vi "Test IODIR Configured as Output on Create.vi"(11 "Test Case In":refnum<class "MCP23017 Test.lvclass">) -> (0 "error out":errorcluster, 3 "Test Case Out":refnum<class "MCP23017 Test.lvclass">)   [LabVIEW 2020, in "MCP23017 Test.lvclass"]
uses:
  MCP23017 Test.lvclass
  C:/Program Files (x86)/National Instruments/LabVIEW 2020/vi.lib/Astemes/LUnit/Test Case.lvclass
  Mock I2C Bus/Mock I2C Bus.lvclass
  C:/Program Files (x86)/National Instruments/LabVIEW 2020/vi.lib/Astemes/LMock/Mock.lvclass
  MCP23017 Test.lvclass/MCP23017 Test.ctl
  <vilib>/Astemes/LMock/One Identical Inputs.vi
  <vilib>/Astemes/LMock/LMock Verifier.lvclass
  <vilib>/Astemes/LMock/LMock.lvlib
  C:/git/astemes-mocking-exercise/tests/Mock I2C Bus/Mock I2C Bus.lvclass
  C:/git/astemes-mocking-exercise/source/I2C Bus Interface/I2C Bus.lvclass
  source/MCP23017/MCP23017.lvclass
  <vilib>/Astemes/LMock/LMock One.lvlib
  C:/Program Files (x86)/National Instruments/LabVIEW 2020/vi.lib/Astemes/LUnit/LUnit Runnable.lvclass
  C:/git/astemes-mocking-exercise/tests/MCP23017 Test/MCP23017 Test.lvclass
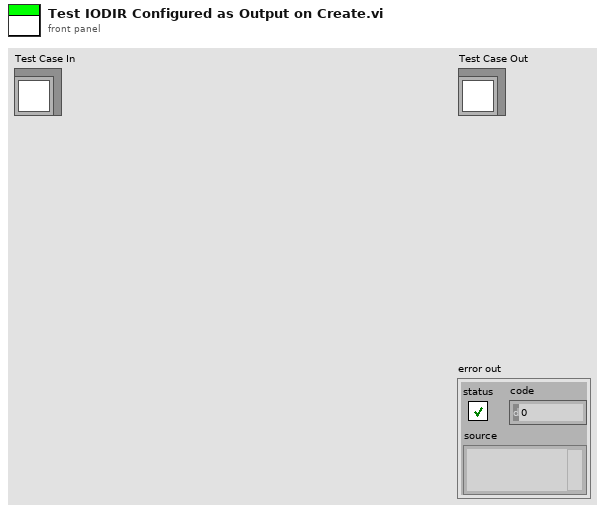
[diagram p1: front panel]
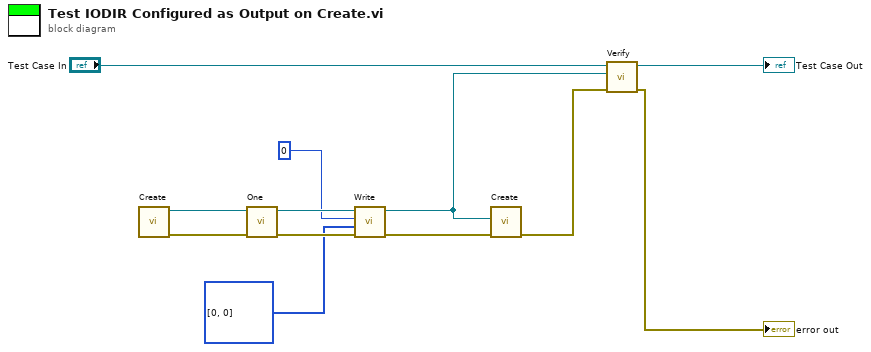
[diagram p0: block diagram]
diagram:
  n1 = call "Create.vi"() -> ("error out"=w9:errorcluster, "Mock Class Generator out"=w7:refnum<class "Mock I2C Bus.lvclass">)  [unwired: 10 in]
  n2 = call-poly <vilib>:"One.vi"("error in (no error)"=w9, "Mock in"=w7) -> ("error out"=w8:errorcluster, "Mock out"=w6:refnum<class "Mock I2C Bus.lvclass">)  [unwired: 8 in]
  n3 = call-dynamic "Write.vi"("error in (no error)"=w8, "Data"=u8[] [0, 0], "Address"=u8 0, "I2C Bus In"=w6) -> ("error out"=w3:errorcluster, "I2C Bus Out"=w1:refnum<class "Mock I2C Bus.lvclass">)  [unwired: 6 in]
  n4 = call "Create.vi"("error in (no error)"=w3, "I2C Bus"=w1) -> ("error out"=w2:errorcluster)  [unwired: 8 in, 1 out]
  n5 = call <vilib>:"Verify.vi"("error in (no error)"=w2, "Mock"=w1, "LUnit Test Case In"="Test Case In") -> ("error out"=→"error out":errorcluster, "LUnit Test Case Out"=→"Test Case Out":refnum<class "MCP23017 Test.lvclass">)  [unwired: 7 in]
